vi "Tx_Create FIFO Association - Acyclic Labels - Trigger Channels.vi"(8 "error in (no error)":errorcluster, 11 "Input Channel Data []":T3[](array[typedef]) {"Labels Settings"."Label Timestamp Channel Data Reference" format="%.0x"; "Labels Settings"."Label Disable/Trigger Channel Reference" format="%.0x"; "Labels Settings"."Word"."Param Setting"."Item Refs" format="%.0x"; "Labels Settings"."Word"."Param Setting"."Num Bits" min=1 max=32; "Labels Settings"."Word"."Param Setting"."Start Bit" min=8 max=31; "Labels Settings"."Label" format="%.0o"}) -> (0 "error out":errorcluster, 3 "Map":T1[](array[typedef]) {"Channel Data Reference" format="%.0x"})   [LabVIEW 2020, in "Ballard Arinc-429 Engine.lvlib"]
doc: "This VI creates a static association between NI-VS FIFO Channel Index and Physical Channel, Label Index for Trigger Channel of an Acyclic Tx Label."
uses:
  Ballard Arinc-429 Engine.lvlib
  Shared/Controls and Global/RT HW Channel.ctl
  Shared/Controls and Global/RT Label Settings.ctl
  Shared/Controls and Global/Label.ctl
  Shared/Controls and Global/transferPeriod.ctl
  Shared/Controls and Global/RT Word Settings.ctl
  Shared/Controls and Global/RT Param Setting.ctl
  Shared/Controls and Global/Start Bit.ctl
  Shared/Controls and Global/Number of Bits.ctl
  <vilib>/NI VeriStand/Custom Device API/Block Data Reference.ctl
  <vilib>/NI VeriStand/Custom Device API/Data Reference.ctl
  <vilib>/NI VeriStand/Custom Device API/Custom Device Item Ref.ctl
  Shared/Controls and Global/TransferType.ctl
  RT Controls/RT Tx Association Trigger Channels.ctl
  <vilib>/NI VeriStand/Custom Device API/Custom Device API.lvlib
  Shared/Ballard Arinc-429 Shared.lvlib
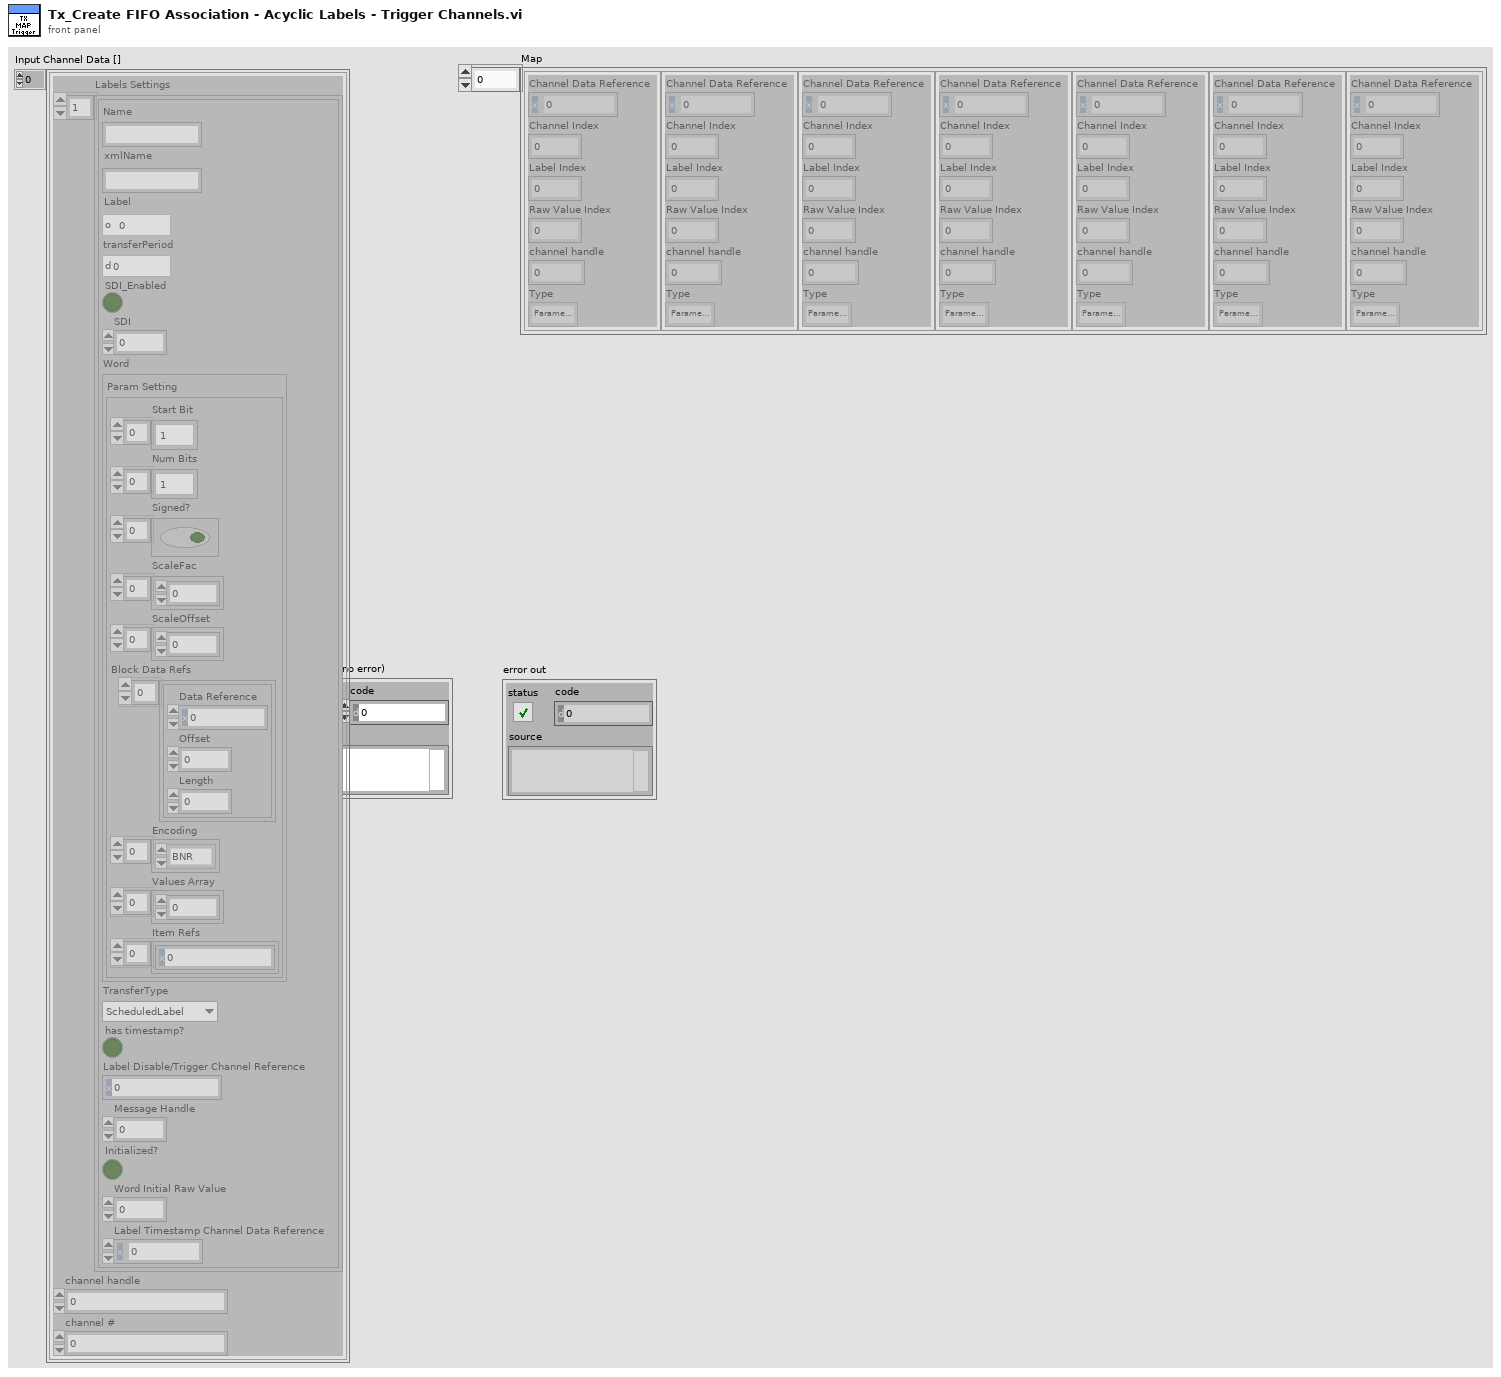
[diagram p1: front panel]
types:
  T1 = typedef "Ballard Arinc-429 Engine.lvlib/RT Tx Association Trigger Channels.ctl" = cluster{"Channel Data Reference":T2, "Channel Index":i32, "Label Index":i32, "Raw Value Index":i32, "channel handle":u64, "Type":enum16{"Parameter Channel", "Disable/Trigger Channel"}}
  T2 = typedef "Custom Device API.lvlib/Data Reference.ctl" = i32
  T3 = typedef "Ballard Arinc-429 Shared.lvlib/RT HW Channel.ctl" = cluster{"Labels Settings":T4[], "channel handle":u64, "channel #":u16}
  T4 = typedef "Ballard Arinc-429 Shared.lvlib/RT Label Settings.ctl" = cluster{"Name":string, "xmlName":string, "Label":T5, "transferPeriod":T6, "SDI_Enabled":bool, "SDI":u8, "Word":T7, "TransferType":T13, "has timestamp?":bool, "Label Disable/Trigger Channel Reference":T12, "Message Handle":u64, "Initialized?":bool, "Word Initial Raw Value":u32, "Label Timestamp Channel Data Reference":T2}
  T5 = typedef "Ballard Arinc-429 Shared.lvlib/Label.ctl" = u8
  T6 = typedef "Ballard Arinc-429 Shared.lvlib/transferPeriod.ctl" = u32
  T7 = typedef "Ballard Arinc-429 Shared.lvlib/RT Word Settings.ctl" = cluster{"Param Setting":T8}
  T8 = typedef "Ballard Arinc-429 Shared.lvlib/RT Param Setting.ctl" = cluster{"Start Bit":T9[], "Num Bits":T10[], "Signed?":bool[], "ScaleFac":dbl[], "ScaleOffset":dbl[], "Block Data Refs":T11[], "Encoding":enum16{"BNR", "BCD", "Discrete"}[], "Values Array":dbl[], "Item Refs":T12[]}
  T9 = typedef "Ballard Arinc-429 Shared.lvlib/Start Bit.ctl" = i32
  T10 = typedef "Ballard Arinc-429 Shared.lvlib/Number of Bits.ctl" = i32
  T11 = typedef "Custom Device API.lvlib/Block Data Reference.ctl" = cluster{"Data Reference":T2, "Offset":u64, "Length":u64}
  T12 = typedef "Custom Device API.lvlib/Custom Device Item Ref.ctl" = u64
  T13 = typedef "Ballard Arinc-429 Shared.lvlib/TransferType.ctl" = enum16{"ScheduledLabel", "Acyclic", "Block", "Strobe"}
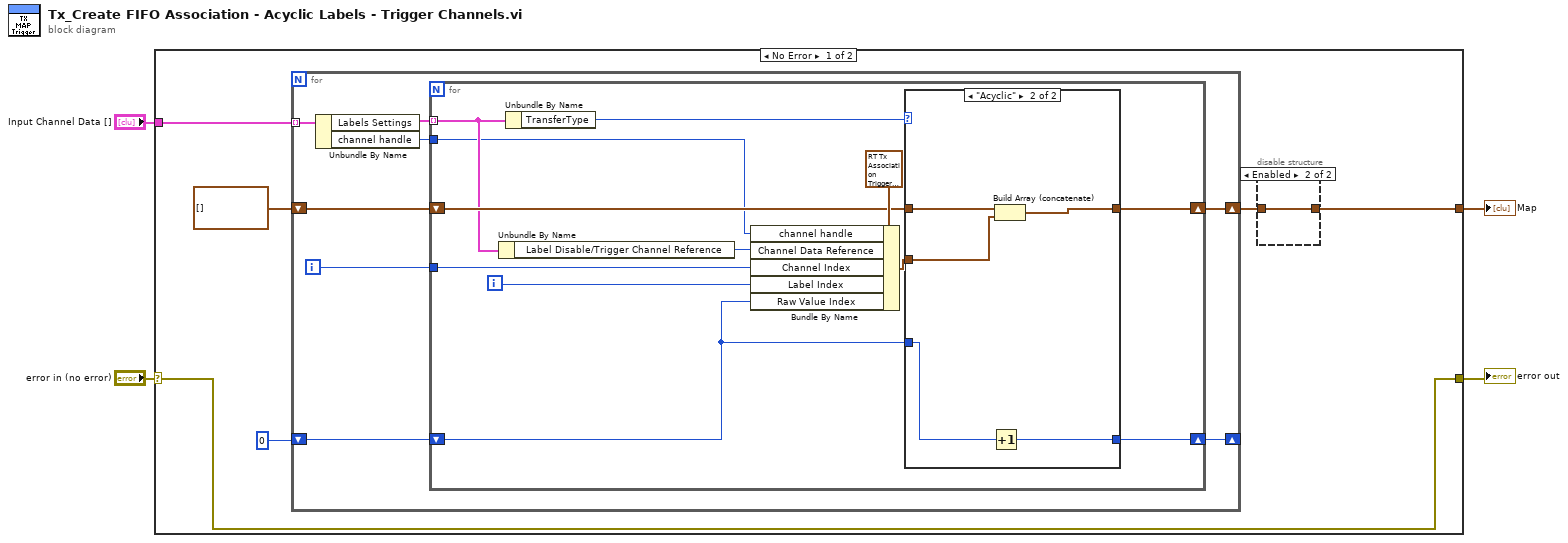
[diagram p0: block diagram]
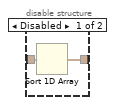
[diagram p2: hidden frame]
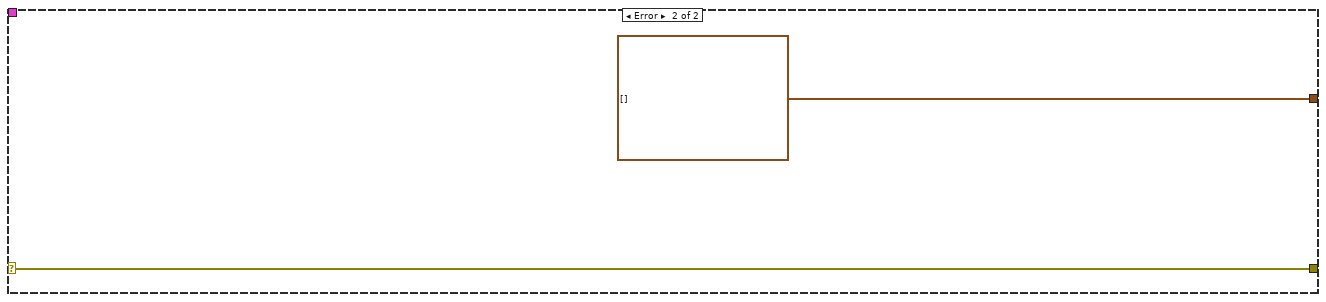
[diagram p4: hidden frame]
diagram:
  n1 = case shown="No Error" "error in (no error)" {
    selector: "error in (no error)" -> [w8 w42]
    tunnel: [w8 w42] -> w3
    tunnel: "Input Channel Data []" -> [w10 _]
    tunnel: [w6 T1[] []] -> w1
    frame No Error {
      n2 = for {
        tunnel: w10 -> [w20] mode=indexing
        shift-right: [w17] -> w7
        shift-left: T1[] [] -> [w19]
        shift-right: [w14] -> _
        shift-left: 0 -> [w16]
        i -> [w18]
        n3 = Unbundle By Name(w20) -> ("Labels Settings"=w21:T4[], "channel handle"=w15:u64)
        n4 = for {
          tunnel: w21 -> [w28] mode=indexing
          shift-right: [w26] -> w17
          shift-left: w19 -> [w31]
          tunnel: w18 -> [w32]
          shift-right: [w22] -> w14
          shift-left: w16 -> [w23]
          tunnel: w15 -> [w24]
          i -> [w29]
          n5 = Unbundle By Name(w28) -> ("Label Disable/Trigger Channel Reference"=w27:T12)
          n6 = Unbundle By Name(w28) -> ("TransferType"=w25:T13)
          n7 = Bundle By Name(cluster=T1 {"Channel Data Reference"=0, "Channel Index"=0, "Label Index"=0, "Raw Value Index"=-1, "channel handle"=0, "Type"=enum."Disable/Trigger Channel"} ("Association"), "channel handle"=w24, "Channel Data Reference"=w27, "Channel Index"=w32, "Label Index"=w29, "Raw Value Index"=w23) -> (w30:T1)
          n8 = case shown="\"Acyclic\"" w25 {
            tunnel: w31 -> [w35 w40]
            tunnel: w30 -> [_ w39]
            tunnel: [w35 w38] -> w26
            tunnel: w23 -> [w34 w37]
            tunnel: [w34 w36] -> w22
            frame "ScheduledLabel", Default {
            }
            frame "Acyclic" {
              n9 = Increment(x=w37) -> (x+1=w36:i32)
              n10 = Build Array (concatenate)(w40, w39) -> (w38:T1[])
            }
          }
        }
      }
      n11 = disable-structure shown="Enabled" {
        disable-tunnel: w7 -> [w12 w13]
        disable-tunnel: [w11 w13] -> w6
        frame Disabled {
          n12 = Sort 1D Array(array=w12) -> (sorted array=w11:T1[])
        }
        frame Enabled {
        }
      }
    }
    frame Error {
    }
  }
  "error out" <- w3
  "Map" <- w1
